vi "PH_Beckhoff.publish analog DIM service.vi"(5 "error in":errorcluster, 6 "Value":dbl, 7 "Quality ok?":bool, 8 "Service ID":i32) -> (0 "error out":errorcluster)   [LabVIEW 2014, in "PH_Beckhoff.lvlib"]
doc: "This VI is used to publish an analog DIM service including quality."
uses:
  PH_Beckhoff.lvlib
  CSlibraries-extern/DimLVEvent/LVDimInterface/LVDimInterface.lvlib
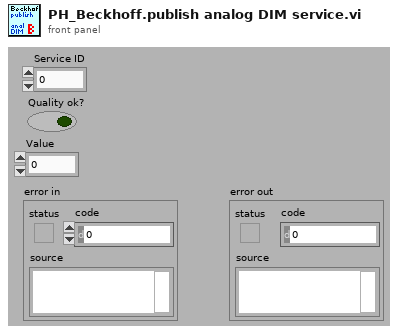
[diagram p1: front panel]
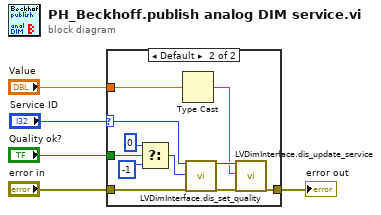
[diagram p0: block diagram]
diagram:
  n1 = case shown="Default" "Service ID" {
    selector: "Service ID" -> [_ w8]
    tunnel: "Quality ok?" -> [_ w14]
    tunnel: "Value" -> [_ w7]
    tunnel: "error in" -> [w6 w10]
    tunnel: [w6 w9] -> w4
    frame -1 {
    }
    frame Default {
      n2 = Select(t=0, s=w14, f=-1) -> (s? t:f=w13:i32)
      n3 = Type Cast(x=w7) -> (*(type *) &x=w15:string)  [unwired: 1 in]
      n4 = call "LVDimInterface.dis_set_quality.vi"("my_serviceID"=w8, "quality"=w13, "error in (no error)"=w10) -> ("my_serviceID (out)"=w16:i32, "error out"=w17:errorcluster)  [unwired: 15 in]
      n5 = call "LVDimInterface.dis_update_service.vi"("my_serviceID"=w16, "data"=w15, "error in (no error)"=w17) -> ("error out"=w9:errorcluster)  [unwired: 14 in, 2 out]
    }
  }
  "error out" <- w4
